vi "correction_data_starter.vi"() -> ()   [LabVIEW 2020]
uses:
  CasaoManagerGeneralSpecifications.ctl
  General dimensions definition.ctl
  Point2D.ctl
  Point2Df.ctl
  WavefrontCorrector.lvclass
  Camera.lvclass
  CorrectionDataManager.lvclass
  Image.lvclass
  InteractionMatrixAcquisitionParameters.ctl
  HasoSlopes.lvclass
  InteractionMatrixToCommandMatrixParameters.ctl
panel:
  in  "init_state_from_config_file":bool
  out "Camera Image (commande 1)":u32[][](graph)
  in  "Start Acq":bool
  out "Camera Image (commande 2)":u32[][](graph)
  in  "number of images to sum":u32=1
  in  "Exposure time (us)":i32=1000
  out "# of valid actuators":u32
  out "Singular values":dbl[](graph)
  in  "Correction data file name":string="Data\\data_correction_manager_example.aoc"
  in  "WavefrontCorrector Configuration file path":path
  out "error out":errorcluster
  out "Informations extracted \nfrom configuration files":T1 caption="Informations extracted from configuration files"
  in  "Haso configuration file path":path
  # "This example is Hardware-dependant, \nplease use your own Haso and corrector configuration file and acquisition system"
  # "Acquisition parameters"
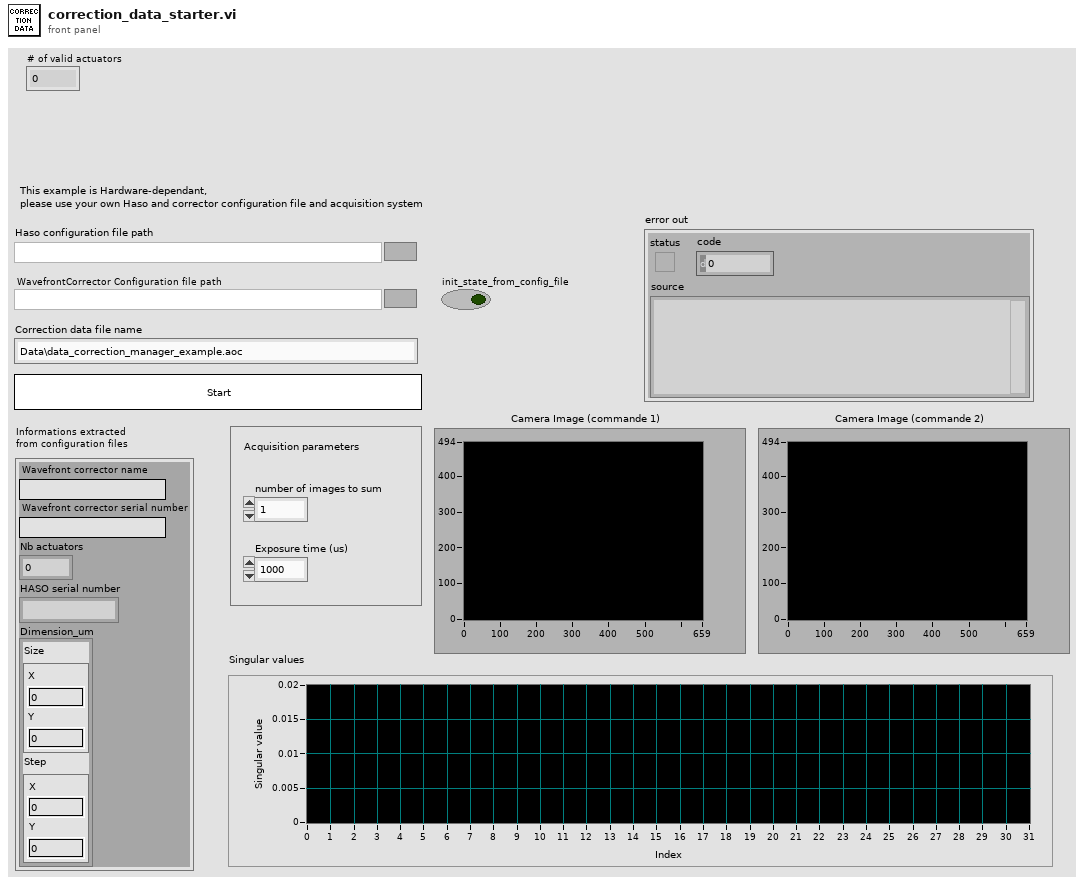
[diagram p1: front panel]
types:
  T1 = typedef "CasaoManagerGeneralSpecifications.ctl" = cluster{"Wavefront corrector name":string, "Wavefront corrector serial number":string, "Nb actuators":i32, "HASO serial number":string, "Dimension_um":T2}
  T2 = typedef "General dimensions definition.ctl" = cluster{"Size":T3, "Step":T4}
  T3 = typedef "Point2D.ctl" = cluster{"X":u32, "Y":u32}
  T4 = typedef "Point2Df.ctl" = cluster{"X":sgl, "Y":sgl}
  T5 = typedef "InteractionMatrixAcquisitionParameters.ctl" = cluster{"Push - Pull value":sgl}
  T6 = typedef "InteractionMatrixToCommandMatrixParameters.ctl" = cluster{"Number of kept modes":i32, "Tilt filtering":bool}
  T7 = typedef "Data alignment enum.ctl" = enum16{"8", "16", "32"}
  T8 = typedef "Wavefront Corrector states - ONE.ctl" = cluster{"Max":sgl, "Min":sgl, "Validity":enum16{"valid", "fixed", "invalid"}, "Fixed_Position":sgl}
  T9 = typedef "HasoSpecifications.ctl" = cluster{"Serial number":string, "Revision":string, "Model":string, "Dimensions_um":T2, "Pixel position for alignment":T4, "Radius tolerance":u16, "Default start subaperture_sspp":T3, "Lower calibration wavelength_nm":dbl, "Upper calibration wavelength_nm":dbl, "Black subaperture position_sspp":T3, "TiltLimit_mrad":dbl, "Radius_m":dbl, "Smearing limit wavelength_nm":dbl, "Smearing limit exposure duration_us":dbl, "Focal_um":dbl}
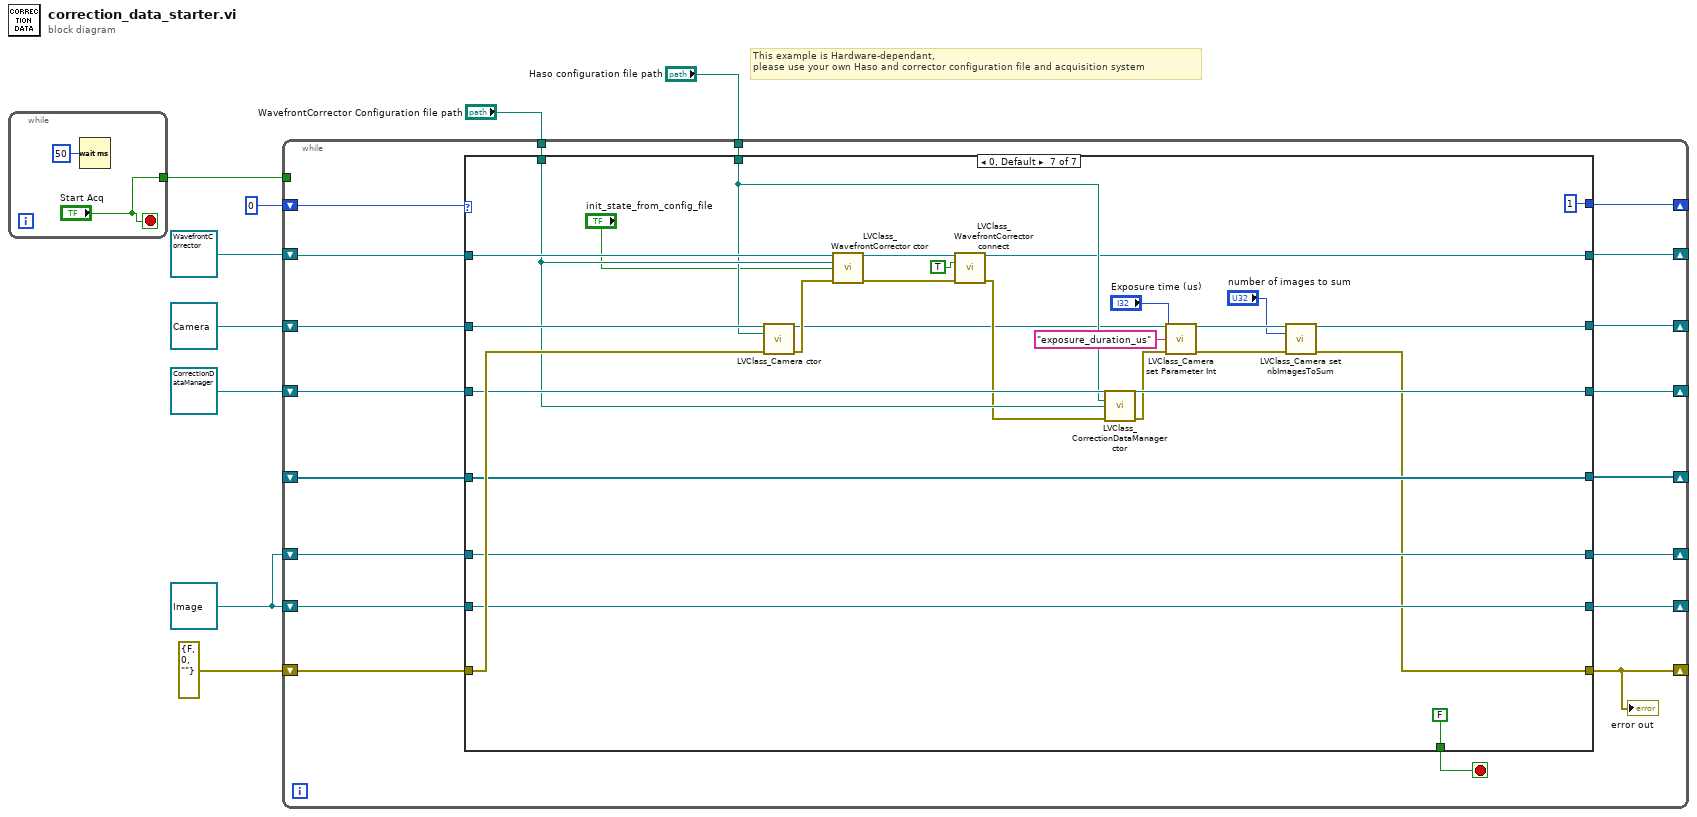
[diagram p0: block diagram]
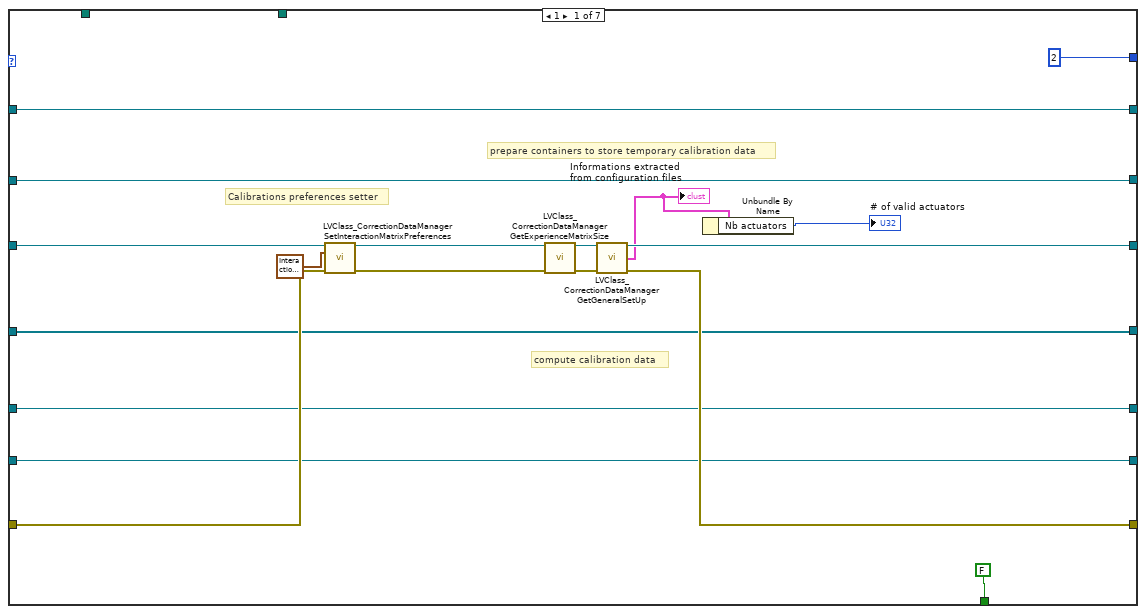
[diagram p2: hidden frame]
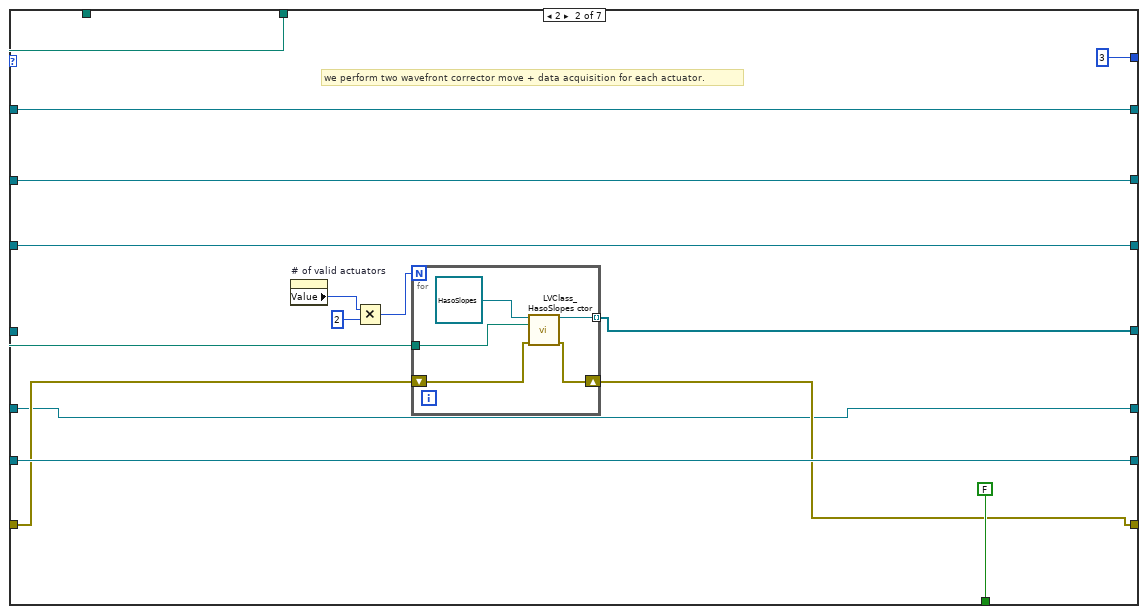
[diagram p3: hidden frame]
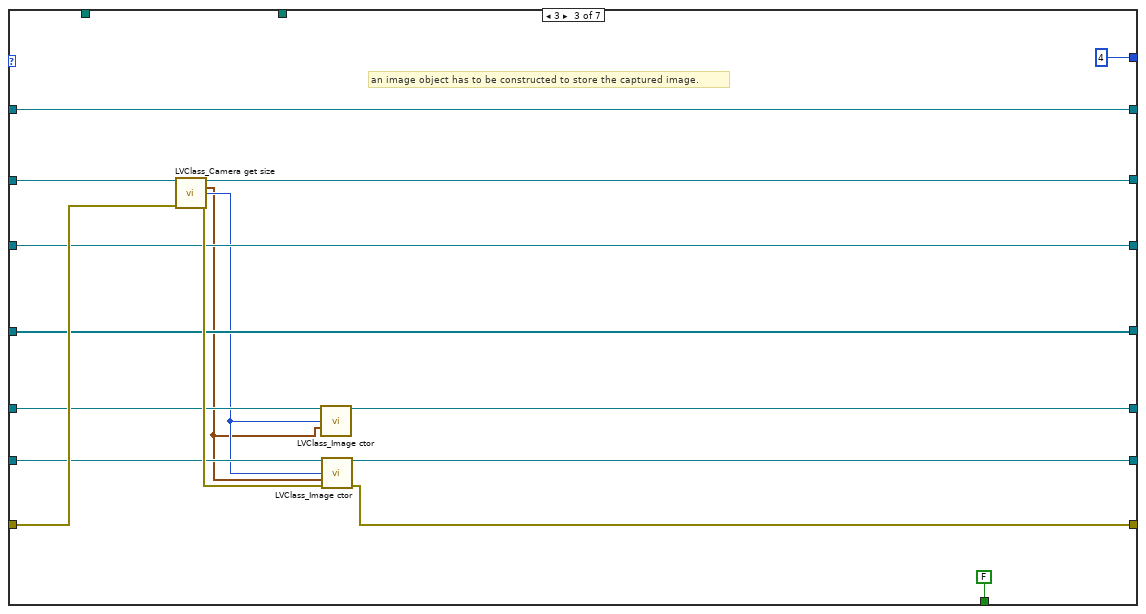
[diagram p4: hidden frame]
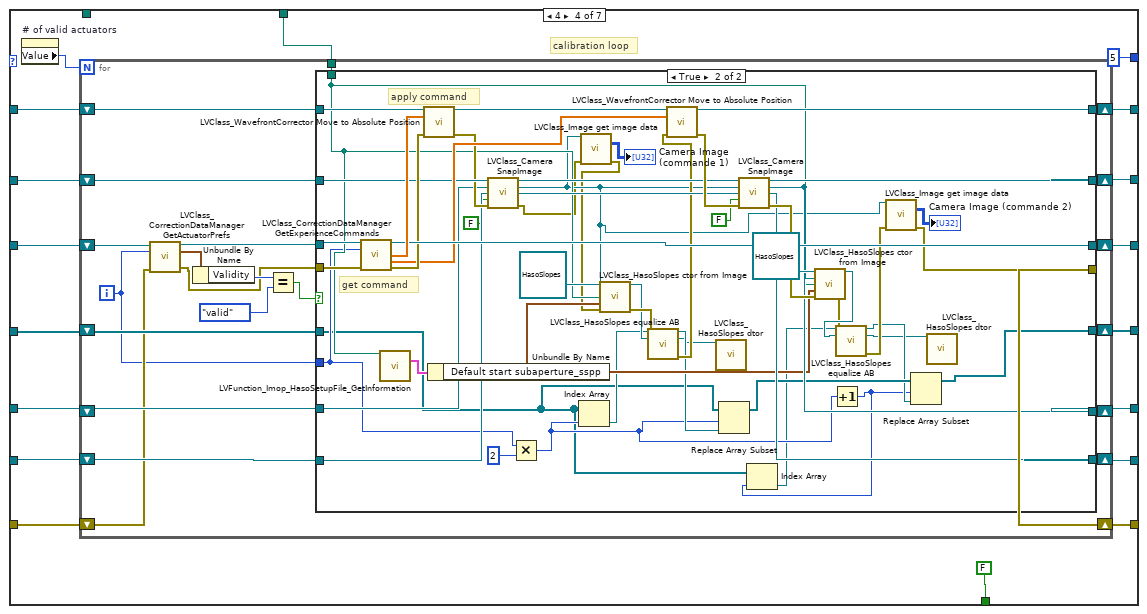
[diagram p5: hidden frame]
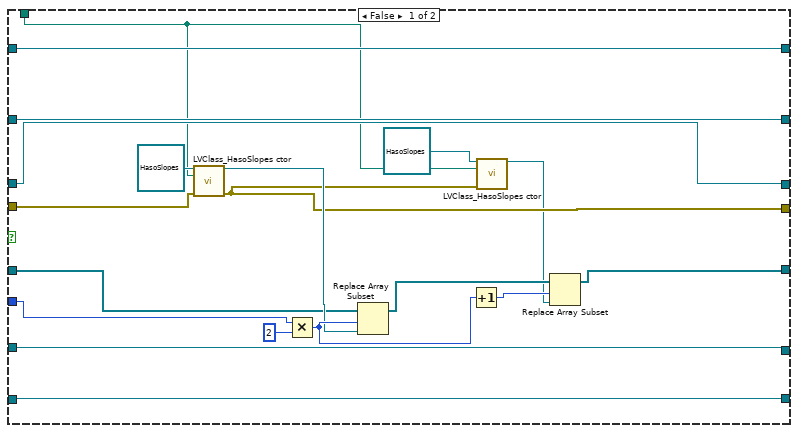
[diagram p6: hidden frame]
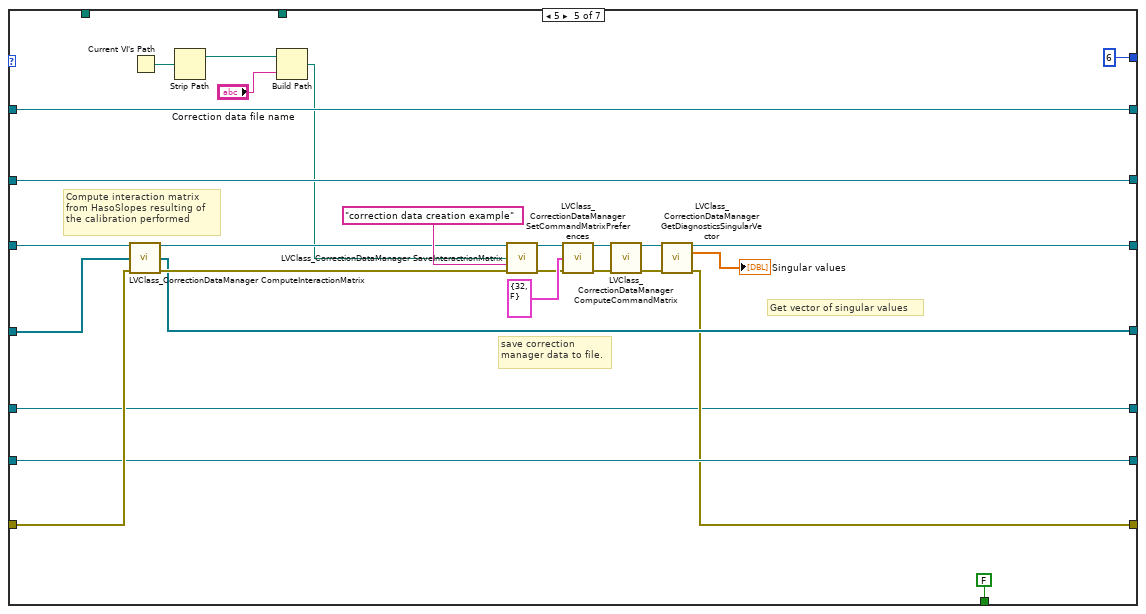
[diagram p7: hidden frame]
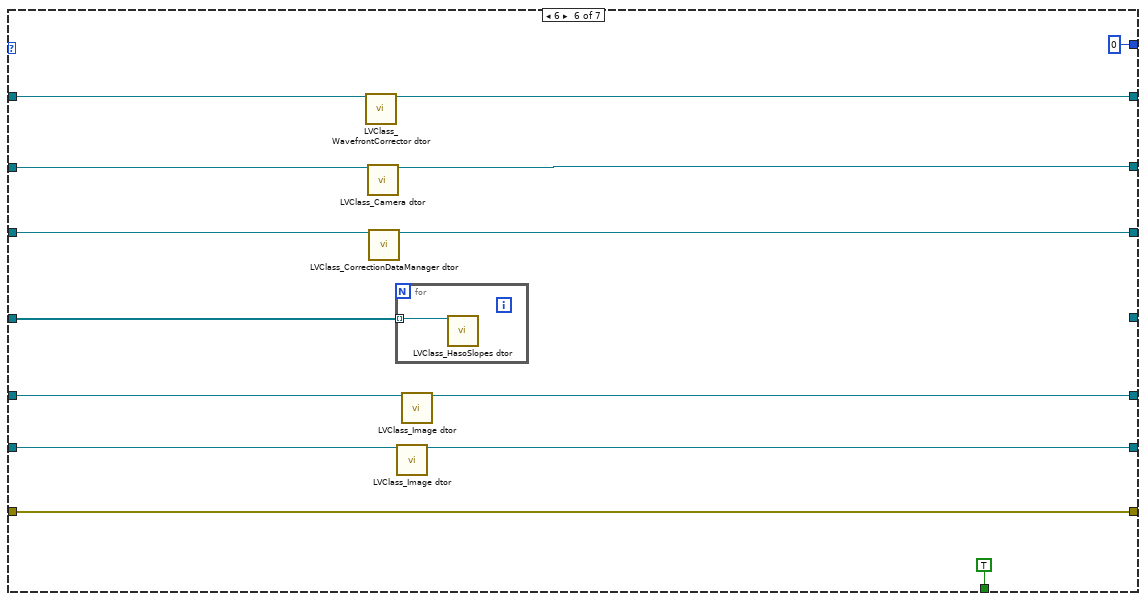
[diagram p8: hidden frame]
diagram:
  w2 = refnum<class "Image.lvclass"> refnum ("Image in")
  # "This example is Hardware-dependant, \nplease use your own Haso and corrector configuration file and acquisition system"
  n1 = while {
    tunnel: ["Start Acq"] -> w1
    stop <- "Start Acq" stop-if-true
    n2 = Wait (ms)(milliseconds to wait=u32 50) -> ()  [unwired: 1 out]
  }
  n3 = while {
    shift-right: [w21] -> _
    shift-left: refnum<class "WavefrontCorrector.lvclass"> refnum ("WavefrontCorrector in") -> [w24]
    shift-right: [w19] -> _
    shift-left: refnum<class "Camera.lvclass"> refnum ("Camera") -> [w27]
    shift-right: [w20] -> _
    shift-left: refnum<class "CorrectionDataManager.lvclass"> refnum ("CorrectionDataManager in") -> [w22]
    shift-right: [w16] -> _
    shift-left: w2 -> [w18]
    shift-right: [w29] -> _
    shift-left: 0 -> [w30]
    shift-right: [w14] -> _
    shift-left: errorcluster {"status"=FALSE, "code"=0, "source"=""} ("error out") -> [w26]
    tunnel: "WavefrontCorrector Configuration file path" -> [w25]
    tunnel: "Haso configuration file path" -> [w23]
    shift-right: [w17] -> _
    shift-left: _ -> [w15]
    shift-right: [w12] -> _
    shift-left: w2 -> [w13]
    tunnel: w1 -> [_]
    stop <- w28 stop-if-true
    n4 = case shown="0, Default" w30 {
      tunnel: [2 3 4 5 6 0 1] -> w29
      tunnel: [FALSE FALSE FALSE FALSE FALSE TRUE FALSE] -> w28
      tunnel: w27 -> [w35 w57 w81 w90 w199 w233 w262]
      tunnel: [w38 w54 w76 w91 w197 w223 w242] -> w14
      tunnel: w26 -> [w42 w53 w80 w98 w217 w223 w261]
      tunnel: w25 -> [_ _ _ _ _ _ w257]
      tunnel: w24 -> [w36 w58 w74 w97 w200 w232 w260]
      tunnel: w23 -> [_ w60 _ w94 _ _ w254]
      tunnel: w22 -> [w43 w56 w73 w99 w219 w229 w259]
      tunnel: [w36 w58 w74 w93 w200 w228 w249] -> w21
      tunnel: [w39 w56 w73 w92 w201 w222 w258] -> w20
      tunnel: [w35 w57 w75 w89 w199 w227 w246] -> w19
      tunnel: w18 -> [w34 w55 w78 w88 w198 w230 w255]
      tunnel: [w37 w59 w72 w95 w203 _ w256] -> w17
      tunnel: [w34 w55 w77 w85 w198 w226 w255] -> w16
      tunnel: w15 -> [w37 _ w72 w96 w218 w231 w256]
      tunnel: w13 -> [w33 w52 w71 w87 w196 w225 w253]
      tunnel: [w33 w52 w68 w86 w196 w224 w253] -> w12
      frame 1 {
        # "prepare containers to store temporary calibration data"
        # "compute calibration data"
        # "Calibrations preferences setter"
        n5 = call "LVClass_CorrectionDataManager SetInteractionMatrixPreferences.vi"("CorrectionDataManager in"=w43, "push_pull_value"=T5 {"Push - Pull value"=0.2} ("Interaction Matrix Parameters 2"), "error in (no error)"=w42) -> ("CorrectionDataManager out"=w44:refnum<class "CorrectionDataManager.lvclass">, "error out"=w45:errorcluster)  [unwired: 11 in]
        n6 = call "LVClass_CorrectionDataManager GetExperienceMatrixSize.vi"("CorrectionDataManager in"=w44, "error in (no error)"=w45) -> ("CorrectionDataManager out"=w41:refnum<class "CorrectionDataManager.lvclass">, "error out"=w40:errorcluster)  [unwired: 10 in, 2 out]
        n7 = call "LVClass_CorrectionDataManager GetGeneralSetUp.vi"("CorrectionDataManager in"=w41, "error in (no error)"=w40) -> ("CorrectionDataManager out"=w39:refnum<class "CorrectionDataManager.lvclass">, "general"=w32:T1, "error out"=w38:errorcluster)  [unwired: 11 in]
        "Informations extracted \nfrom configuration files" <- w32
        n8 = Unbundle By Name(w32) -> ("Nb actuators"=→"# of valid actuators":i32)
      }
      frame 2 {
        # "we perform two wavefront corrector move + data acquisition for each actuator."
        n9 = property on="# of valid actuators" class="DigNum (strict)"() -> ("Value"=w50:u32)  [unwired: 2 in, 2 out]
        n10 = Multiply(x=w50, y=u32 2) -> (x*y=w49:u32)
        n11 = for {
          N: w49 -> [_]
          tunnel: w60 -> [w67]
          tunnel: [w65] -> w59 mode=indexing
          shift-right: [w64] -> w54
          shift-left: w53 -> [w63]
          n12 = call "LVClass_HasoSlopes ctor.vi"("HasoSlopes (const)"=refnum<class "HasoSlopes.lvclass"> refnum ("HasoSlopes in"), "Configuration file path"=w67, "error in (no error)"=w63) -> ("HasoSlopes (new)"=w65:refnum<class "HasoSlopes.lvclass">, "error out"=w64:errorcluster)  [unwired: 11 in]
        }
      }
      frame 3 {
        # "an image object has to be constructed to store the captured image."
        n13 = call "LVClass_Camera get size.vi"("Camera in"=w81, "error in (no error)"=w80) -> ("Camera out"=w75:refnum<class "Camera.lvclass">, "size"=w69:T3, "Number of bits"=w70:T7, "error out"=w79:errorcluster)  [unwired: 10 in]
        n14 = call "LVClass_Image ctor.vi"("Image (const)"=w71, "Data alignment"=w70, "Size"=w69) -> ("Image (new)"=w68:refnum<class "Image.lvclass">)  [unwired: 11 in, 1 out]
        n15 = call "LVClass_Image ctor.vi"("Image (const)"=w78, "Data alignment"=w70, "Size"=w69, "error in (no error)"=w79) -> ("Image (new)"=w77:refnum<class "Image.lvclass">, "error out"=w76:errorcluster)  [unwired: 10 in]
      }
      frame 4 {
        # "calibration loop"
        n16 = property on="# of valid actuators" class="DigNum (strict)"() -> ("Value"=w84:u32)  [unwired: 2 in, 2 out]
        n17 = for {
          N: w84 -> [_]
          shift-right: [w122] -> w92
          shift-left: w99 -> [w121]
          shift-right: [w116] -> w93
          shift-left: w97 -> [w123]
          tunnel: w94 -> [w117]
          shift-right: [w115] -> w91
          shift-left: w98 -> [w108]
          shift-right: [w113] -> w89
          shift-left: w90 -> [w114]
          shift-right: [w110] -> w86
          shift-left: w87 -> [w111]
          shift-right: [w109] -> w85
          shift-left: w88 -> [w112]
          shift-right: [w118] -> w95
          shift-left: w96 -> [w119]
          i -> [w102]
          n18 = call "LVClass_CorrectionDataManager GetActuatorPrefs.vi"("CorrectionDataManager in"=w121, "N° actuator"=w102, "error in (no error)"=w108) -> ("CorrectionDataManager out"=w120:refnum<class "CorrectionDataManager.lvclass">, "Actuator state"=w107:T8, "error out"=w103:errorcluster)  [unwired: 10 in]
          n19 = Unbundle By Name(w107) -> ("Validity"=w106:enum16{"valid", "fixed", "invalid"})
          n20 = Equal?(x=w106, y=enum16{"valid", "fixed", "invalid"}."valid" ("Validity")) -> (x = y?=w104:bool)
          n21 = case shown="True" w104 {
            tunnel: w123 -> [w141 w194]
            tunnel: [w142 w192] -> w122
            tunnel: w102 -> [w124 w152]
            tunnel: w120 -> [w142 w191]
            tunnel: w119 -> [w125 w148]
            tunnel: [w126 w157] -> w118
            tunnel: w117 -> [w130 w163]
            tunnel: [w141 w182] -> w116
            tunnel: [w129 w164] -> w115
            tunnel: w114 -> [w140 w181]
            tunnel: [w140 w176] -> w113
            tunnel: w112 -> [w138 w174]
            tunnel: w111 -> [w139 w175]
            tunnel: [w139 w167] -> w110
            tunnel: [w138 w170] -> w109
            tunnel: w103 -> [w133 w169]
            frame False {
              n22 = call "LVClass_HasoSlopes ctor.vi"("HasoSlopes (const)"=refnum<class "HasoSlopes.lvclass"> refnum ("HasoSlopes in"), "Configuration file path"=w130, "error in (no error)"=w133) -> ("HasoSlopes (new)"=w132:refnum<class "HasoSlopes.lvclass">, "error out"=w129:errorcluster)  [unwired: 11 in]
              n23 = Multiply(x=w124, y=2) -> (x*y=w135:i32)
              n24 = Replace Array Subset(array=w125, new element=w132, index=w135) -> (w128:refnum<class "HasoSlopes.lvclass">[])
              n25 = Increment(x=w135) -> (x+1=w137:i32)
              n26 = call "LVClass_HasoSlopes ctor.vi"("HasoSlopes (const)"=refnum<class "HasoSlopes.lvclass"> refnum ("HasoSlopes in"), "Configuration file path"=w130, "error in (no error)"=w129) -> ("HasoSlopes (new)"=w127:refnum<class "HasoSlopes.lvclass">)  [unwired: 11 in, 1 out]
              n27 = Replace Array Subset(array=w128, new element=w127, index=w137) -> (w126:refnum<class "HasoSlopes.lvclass">[])
            }
            frame True {
              # "apply command"
              # "get command"
              n28 = call "LVClass_CorrectionDataManager GetExperienceCommands.vi"("CorrectionDataManager in"=w191, "N° actuator"=w152, "error in (no error)"=w169) -> ("CorrectionDataManager out"=w192:refnum<class "CorrectionDataManager.lvclass">, "First DeltaCommand"=w193:sgl[], "Second DeltaCommand"=w186:sgl[], "error out"=w190:errorcluster)  [unwired: 9 in]
              n29 = call "LVFunction_Imop_HasoSetupFile_GetInformation.vi"("WFS_setup_file IN"=w163) -> ("HASO specifications"=w162:T9)  [unwired: 10 in, 4 out]
              n30 = call "LVClass_WavefrontCorrector Move to Absolute Position.vi"("WavefrontCorrector in"=w194, "Absolute Positions"=w193, "error in (no error)"=w190) -> ("WavefrontCorrector out"=w187:refnum<class "WavefrontCorrector.lvclass">, "error out"=w180:errorcluster)  [unwired: 11 in]
              n31 = Unbundle By Name(w162) -> ("Default start subaperture_sspp"=w161:T3)
              n32 = call "LVClass_Camera SnapImage.vi"("Camera in"=w181, "Image"=w175, "Image RAW"=w174, "remove_background"=FALSE, "error in (no error)"=w180) -> ("Camera out"=w177:refnum<class "Camera.lvclass">, "Image (dup)"=w145:refnum<class "Image.lvclass">, "Image (dup) RAW"=w172:refnum<class "Image.lvclass">, "error out"=w144:errorcluster)  [unwired: 7 in]
              n33 = Multiply(x=w152, y=2) -> (x*y=w151:i32)
              n34 = Index Array(array=w148, index=w151) -> (element=w150:refnum<class "HasoSlopes.lvclass">)
              n35 = call "LVClass_Image get image data.vi"("Image in"=w145, "error in (no error)"=w144) -> ("Image data out"=→"Camera Image (commande 1)":u32[][], "error out"=w143:errorcluster)  [unwired: 11 in, 1 out]
              n36 = call "LVClass_HasoSlopes ctor from Image.vi"("HasoSlopes (const)"=refnum<class "HasoSlopes.lvclass"> refnum ("HasoSlopes in"), "Image"=w145, "Haso configuration file"=w163, "start subpupil"=w161, "error in (no error)"=w143) -> ("HasoSlopes (new)"=w155:refnum<class "HasoSlopes.lvclass">, "error out"=w189:errorcluster)  [unwired: 8 in, 1 out]
              n37 = call "LVClass_HasoSlopes equalize AB.vi"("HasoSlopes dest in"=w150, "HasoSlopes source in"=w155, "error in (no error)"=w189) -> ("HasoSlopes dest out"=w160:refnum<class "HasoSlopes.lvclass">, "HasoSlopes source out"=w154:refnum<class "HasoSlopes.lvclass">, "error out"=w168:errorcluster)  [unwired: 10 in]
              n38 = call "LVClass_WavefrontCorrector Move to Absolute Position.vi"("WavefrontCorrector in"=w187, "Absolute Positions"=w186, "error in (no error)"=w168) -> ("WavefrontCorrector out"=w182:refnum<class "WavefrontCorrector.lvclass">, "error out"=w179:errorcluster)  [unwired: 11 in]
              n39 = call "LVClass_HasoSlopes dtor.vi"("HasoSlopes in"=w154) -> ()  [unwired: 13 in, 2 out]
              n40 = Replace Array Subset(array=w148, new element=w160, index=w151) -> (w159:refnum<class "HasoSlopes.lvclass">[])
              n41 = call "LVClass_Camera SnapImage.vi"("Camera in"=w177, "Image"=w145, "Image RAW"=w172, "remove_background"=FALSE, "error in (no error)"=w179) -> ("Camera out"=w176:refnum<class "Camera.lvclass">, "Image (dup)"=w167:refnum<class "Image.lvclass">, "Image (dup) RAW"=w170:refnum<class "Image.lvclass">, "error out"=w178:errorcluster)  [unwired: 7 in]
              n42 = call "LVClass_HasoSlopes ctor from Image.vi"("HasoSlopes (const)"=refnum<class "HasoSlopes.lvclass"> refnum ("HasoSlopes in"), "Image"=w167, "Haso configuration file"=w163, "start subpupil"=w161, "error in (no error)"=w178) -> ("HasoSlopes (new)"=w185:refnum<class "HasoSlopes.lvclass">, "error out"=w183:errorcluster)  [unwired: 8 in, 1 out]
              n43 = Increment(x=w151) -> (x+1=w149:i32)
              n44 = Index Array(array=w148, index=w149) -> (element=w147:refnum<class "HasoSlopes.lvclass">)
              n45 = call "LVClass_HasoSlopes equalize AB.vi"("HasoSlopes dest in"=w147, "HasoSlopes source in"=w185, "error in (no error)"=w183) -> ("HasoSlopes dest out"=w158:refnum<class "HasoSlopes.lvclass">, "HasoSlopes source out"=w153:refnum<class "HasoSlopes.lvclass">, "error out"=w165:errorcluster)  [unwired: 10 in]
              n46 = call "LVClass_Image get image data.vi"("Image in"=w145, "error in (no error)"=w165) -> ("Image data out"=→"Camera Image (commande 2)":u32[][], "error out"=w164:errorcluster)  [unwired: 11 in, 1 out]
              n47 = Replace Array Subset(array=w159, new element=w158, index=w149) -> (w157:refnum<class "HasoSlopes.lvclass">[])
              n48 = call "LVClass_HasoSlopes dtor.vi"("HasoSlopes in"=w153) -> ()  [unwired: 13 in, 2 out]
            }
          }
        }
      }
      frame 5 {
        # "Get vector of singular values"
        # "save correction\nmanager data to file."
        # "Compute interaction matrix\nfrom HasoSlopes resulting of\nthe calibration performed"
        n49 = call "LVClass_CorrectionDataManager ComputeInteractionMatrix.vi"("CorrectionDataManager in"=w219, "HasoSlopes array"=w218, "error in (no error)"=w217) -> ("CorrectionDataManager out"=w208:refnum<class "CorrectionDataManager.lvclass">, "HasoSlopes array 2"=w203:refnum<class "HasoSlopes.lvclass">[], "error out"=w204:errorcluster)  [unwired: 10 in]
        n50 = Current VI's Path() -> (path=w207:path)
        n51 = Strip Path(path=w207) -> (stripped path=w205:path)  [unwired: 1 out]
        n52 = Build Path(base path=w205, name or relative path="Correction data file name") -> (appended path=w195:path)
        n53 = call "LVClass_CorrectionDataManager SaveInteractrionMatrix.vi"("CorrectionDataManager in"=w208, "Interaction Matrix file path"=w195, "comment"="correction data creation example", "error in (no error)"=w204) -> ("CorrectionDataManager out"=w212:refnum<class "CorrectionDataManager.lvclass">, "error out"=w209:errorcluster)  [unwired: 10 in]
        n54 = call "LVClass_CorrectionDataManager SetCommandMatrixPreferences.vi"("CorrectionDataManager in"=w212, "Prefs"=T6 {"Number of kept modes"=32, "Tilt filtering"=FALSE}, "error in (no error)"=w209) -> ("CorrectionDataManager out"=w213:refnum<class "CorrectionDataManager.lvclass">, "error out"=w216:errorcluster)  [unwired: 11 in]
        n55 = call "LVClass_CorrectionDataManager ComputeCommandMatrix.vi"("CorrectionDataManager in"=w213, "error in (no error)"=w216) -> ("CorrectionDataManager out"=w214:refnum<class "CorrectionDataManager.lvclass">, "error out"=w215:errorcluster)  [unwired: 12 in]
        n56 = call "LVClass_CorrectionDataManager GetDiagnosticsSingularVector.vi"("CorrectionDataManager in"=w214, "error in (no error)"=w215) -> ("CorrectionDataManager out"=w201:refnum<class "CorrectionDataManager.lvclass">, "ArrayOfSingularValues"=→"Singular values":dbl[], "error out"=w197:errorcluster)  [unwired: 11 in]
      }
      frame 6 {
        n57 = call "LVClass_WavefrontCorrector dtor.vi"("WavefrontCorrector in"=w232) -> ("WavefrontCorrector out"=w228:refnum<class "WavefrontCorrector.lvclass">)  [unwired: 13 in, 1 out]
        n58 = call "LVClass_Camera dtor.vi"("Camera in"=w233) -> ("Camera out"=w227:refnum<class "Camera.lvclass">)  [unwired: 13 in, 1 out]
        n59 = call "LVClass_CorrectionDataManager dtor.vi"("CorrectionDataManager in"=w229) -> ("CorrectionDataManager out"=w222:refnum<class "CorrectionDataManager.lvclass">)  [unwired: 13 in, 1 out]
        n60 = for {
          tunnel: w231 -> [w236] mode=indexing
          n61 = call "LVClass_HasoSlopes dtor.vi"("HasoSlopes in"=w236) -> ()  [unwired: 13 in, 2 out]
        }
        n62 = call "LVClass_Image dtor.vi"("Image in"=w230) -> ("Image out"=w226:refnum<class "Image.lvclass">)  [unwired: 13 in, 1 out]
        n63 = call "LVClass_Image dtor.vi"("Image in"=w225) -> ("Image out"=w224:refnum<class "Image.lvclass">)  [unwired: 13 in, 1 out]
      }
      frame 0, Default {
        n64 = call "LVClass_Camera ctor.vi"("Camera (const)"=w262, "Configuration file path"=w254, "error in (no error)"=w261) -> ("Camera (new)"=w238:refnum<class "Camera.lvclass">, "error out"=w252:errorcluster)  [unwired: 11 in]
        n65 = call "LVClass_WavefrontCorrector ctor.vi"("WavefrontCorrector (const)"=w260, "PathToWavefrontCorrectorSetupFile"=w257, "init_state_from_config_file"="init_state_from_config_file", "error in (no error)"=w252) -> ("WavefrontCorrector (new)"=w250:refnum<class "WavefrontCorrector.lvclass">, "error out"=w248:errorcluster)  [unwired: 10 in]
        n66 = call "LVClass_WavefrontCorrector connect.vi"("WavefrontCorrector in"=w250, "set_init_state_from_config_file"=TRUE, "error in (no error)"=w248) -> ("WavefrontCorrector out"=w249:refnum<class "WavefrontCorrector.lvclass">, "error out"=w245:errorcluster)  [unwired: 11 in]
        n67 = call "LVClass_CorrectionDataManager ctor.vi"("CorrectionDataManager (const)"=w259, "PathTohaso_config_file_path"=w254, "PathTowfc_config_file_path"=w257, "error in (no error)"=w245) -> ("CorrectionDataManager (new)"=w258:refnum<class "CorrectionDataManager.lvclass">, "error out"=w243:errorcluster)  [unwired: 10 in]
        n68 = call "LVClass_Camera set Parameter Int.vi"("Camera in"=w238, "parameter_name"="exposure_duration_us", "value"="Exposure time (us)", "error in (no error)"=w243) -> ("Camera out"=w247:refnum<class "Camera.lvclass">, "error out"=w244:errorcluster)  [unwired: 10 in]
        n69 = call "LVClass_Camera set nbImagesToSum.vi"("Camera in"=w247, "nb_image"="number of images to sum", "error in (no error)"=w244) -> ("Camera out"=w246:refnum<class "Camera.lvclass">, "error out"=w242:errorcluster)  [unwired: 11 in]
      }
    }
    "error out" <- w14
  }
